vi "step.util.flag-matching.vi"(6 "include step flags":bool=TRUE, 9 "stepElement":variant, 10 "procElement":variant, 11 "$string in":string="$module $proc $step $clk $date_$time ") -> (3 "formated string out":string="myModule myProc myStep 3800935574.524293 2024-06-11_10-26-15 ")   [LabVIEW 2024]
uses:
  controls/typeProcVarientName.ctl
  controls/typeStepVarients.ctl
  Polymorphics/variantCtrlString.vi
  Polymorphics/variantCtrlNumber.vi
  proc.util.validateParamExist.vi
  <vilib>/Utility/error.llb/Clear Errors.vi
  <vilib>/Utility/error.llb/Trim Whitespace One-Sided.vi
  globals/globals-engine.vi
  util.error.create.vi
  <vilib>/Utility/libraryn.llb/Create Directory Recursive.vi
panel:
  out "array out":string[](array[string])
  in  "time stamp":timestamp
  # "this vi should support matching fields file and io node names"
  # "$date\n$timestamp"
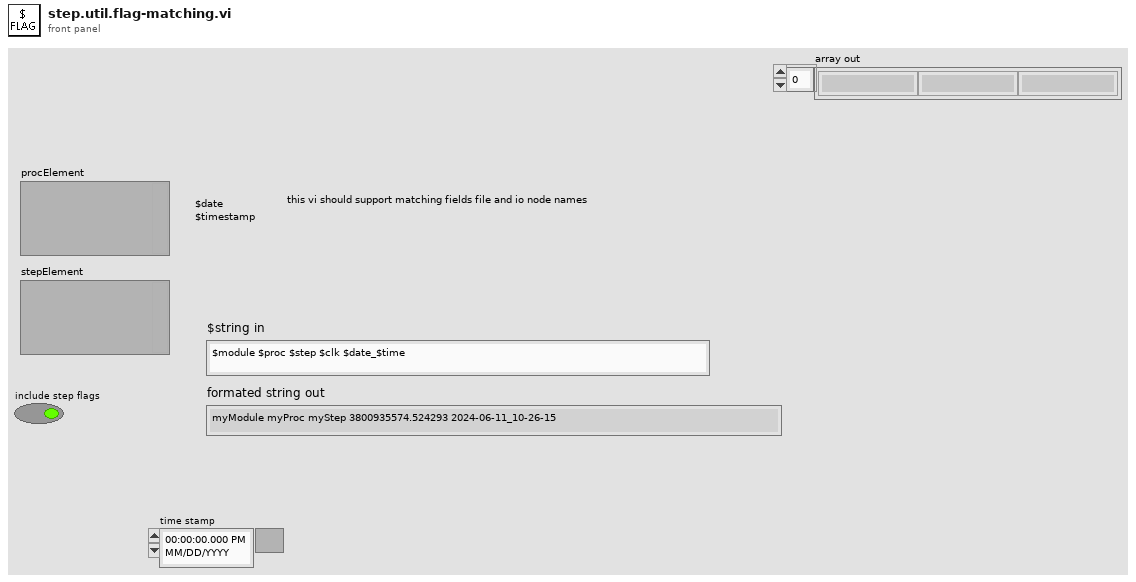
[diagram p1: front panel]
types:
  T1 = typedef "typeStepVarients.ctl" = enum16{"stepNameID", "stepFunction", "stepReport", "stepSetpoint", "stepPointer", "stepProcPointer", "stepIoPointer", "stepIoValue", "stepFilePointer", "stepMessage", "stepTimeString", "stepNumReg", "stepStrReg", "stepSeconds", "stepUnitDoseParams", "stepUnitIndex"}
  T2 = typedef "typeProcVarientName.ctl" = enum16{"procNameID", "procModuleID", "procPath", "procIsRunning", "procIndex", "procModule", "procRegisterNumeric", "procRegisterString", "procReport", "procReportPrev", "procCLK", "procStepPointer", "procType"}
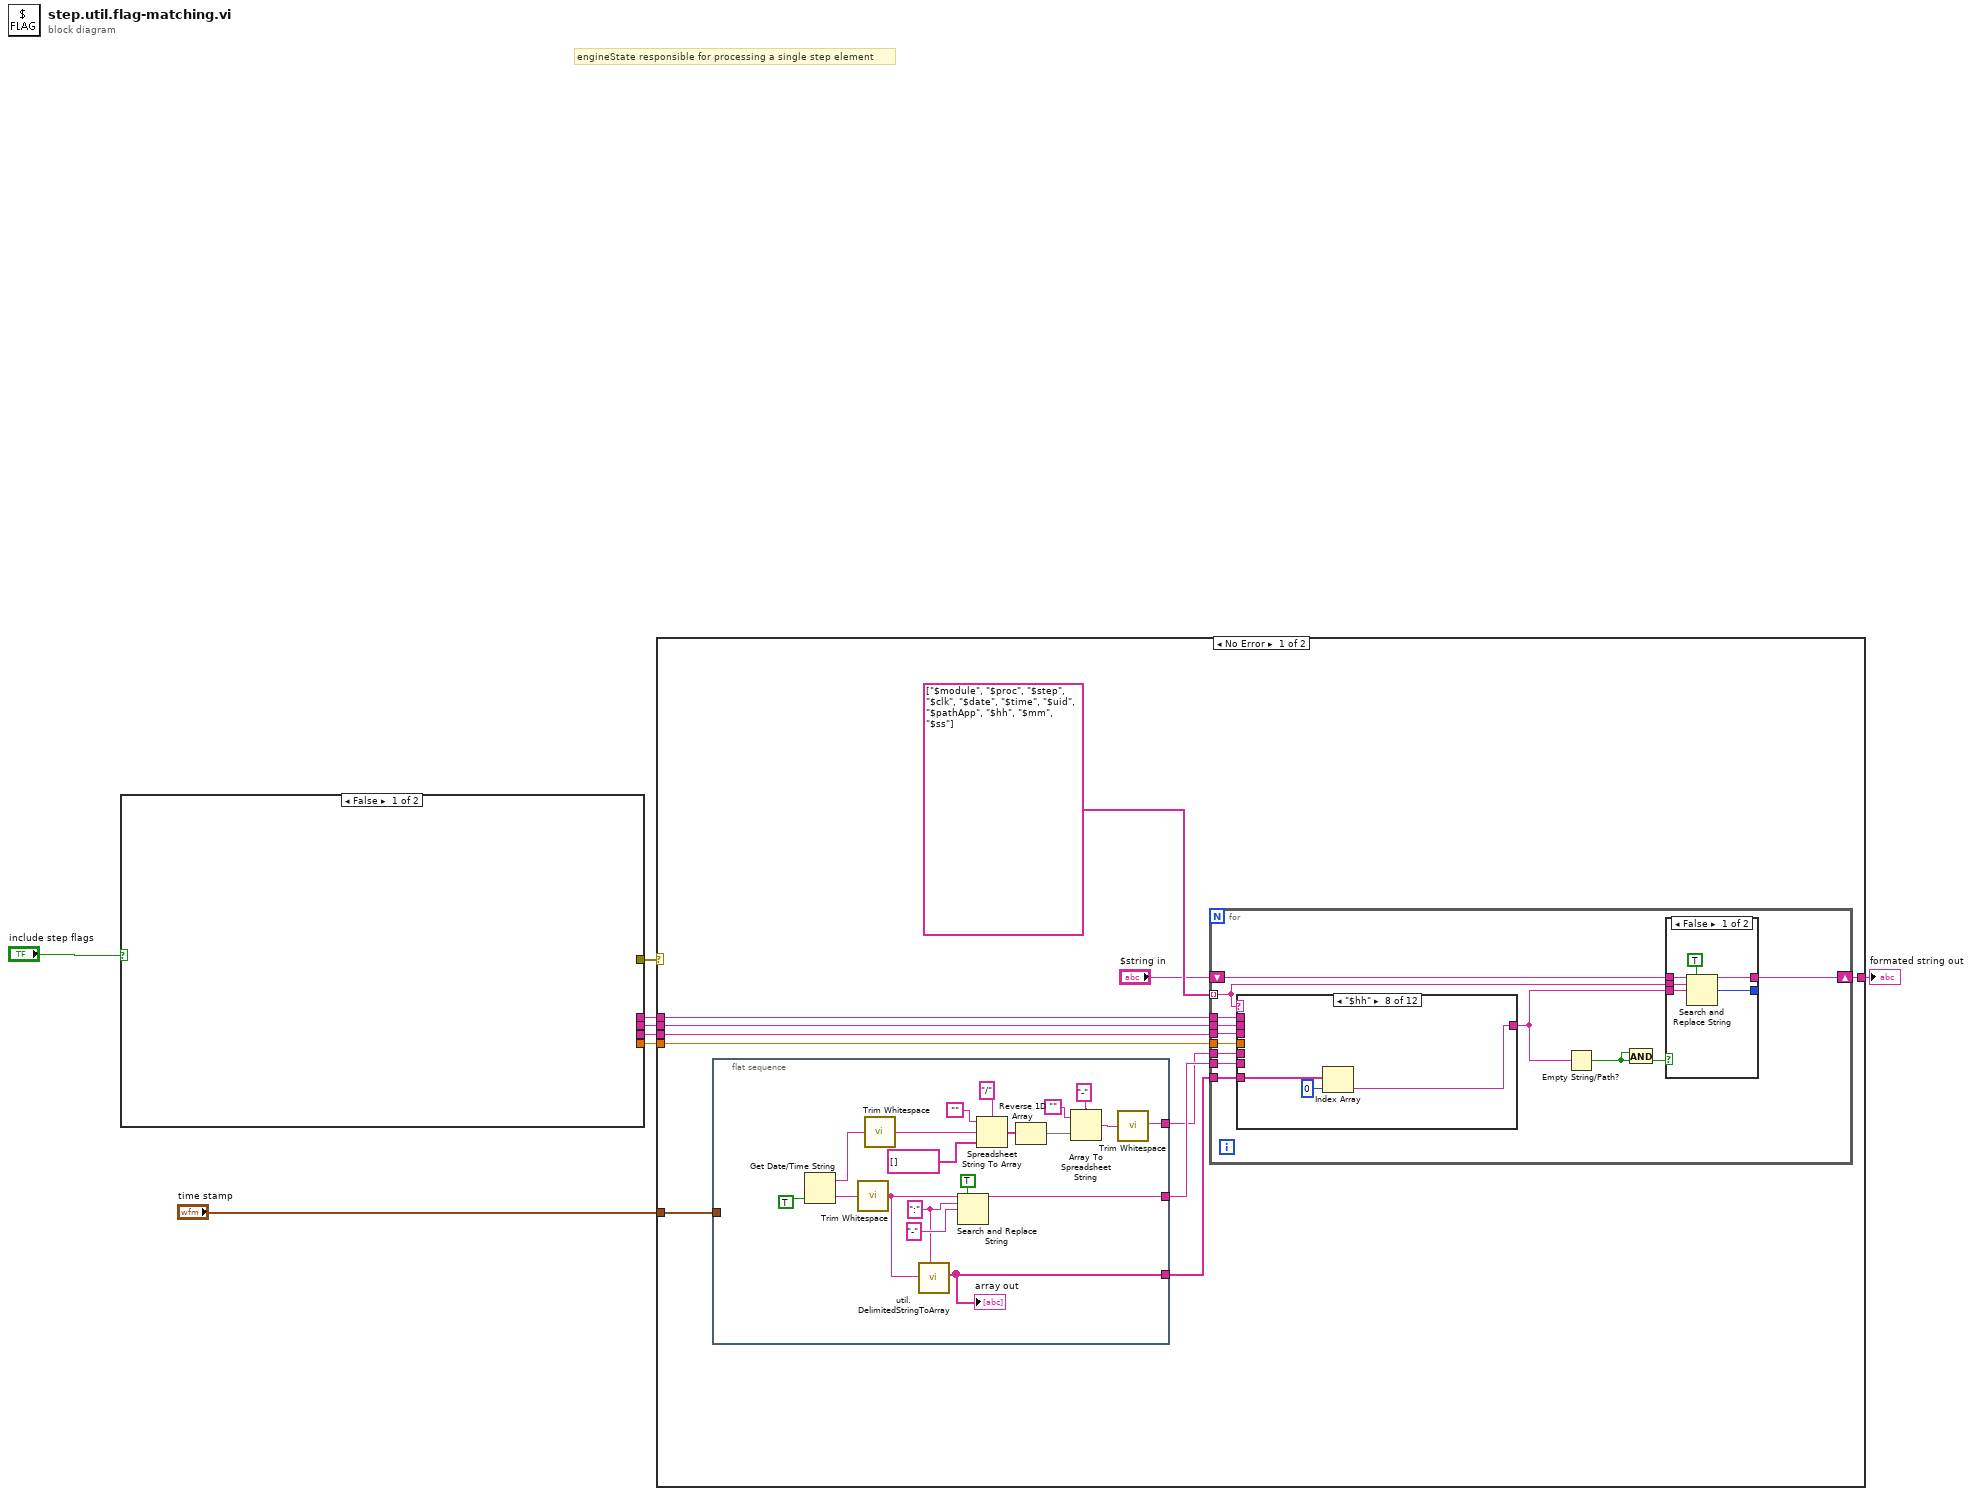
[diagram p0: block diagram]
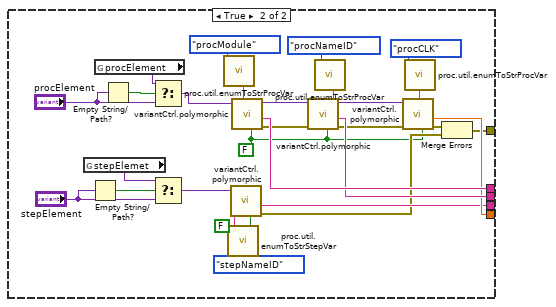
[diagram p2: hidden frame]
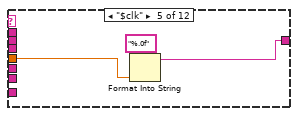
[diagram p8: hidden frame]
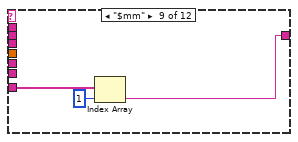
[diagram p11: hidden frame]
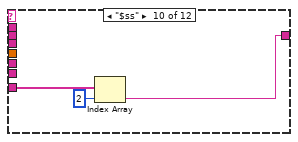
[diagram p12: hidden frame]
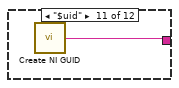
[diagram p13: hidden frame]
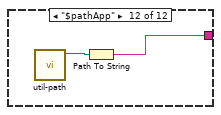
[diagram p14: hidden frame]
diagram:
  # "engineState responsible for processing a single step element"
  n1 = case shown="False" "include step flags" {
    tunnel: [_ w25] -> w7
    tunnel: [_ w24] -> w6
    tunnel: [_ w23] -> w5
    tunnel: [_ w20] -> w4
    tunnel: [_ w11] -> w3
    frame False {
    }
    frame True {
      w9 = FALSE ("isRequired (T)")
      n2 = global read "globals-engine.vi" "stepElemet"() -> (w36:variant)
      n3 = Empty String/Path?(string/path="stepElement") -> (empty?=w15:bool)
      n4 = global read "globals-engine.vi" "procElement"() -> (w37:variant)
      n5 = Empty String/Path?(string/path="procElement") -> (empty?=w17:bool)
      n6 = Select(t=w37, s=w17, f="procElement") -> (s? t:f=w33:variant)
      n7 = Select(t=w36, s=w15, f="stepElement") -> (s? t:f=w35:variant)
      n8 = call "proc.util.enumToStrProcVar.vi"("Proc var"=typeProcVarientName."procModule" ("proc var")) -> ("String"=w31:string)  [unwired: 10 in]
      n9 = call "proc.util.enumToStrStepVar.vi"("Step var"=typeStepVarients."stepNameID" ("proc var")) -> ("String"=w22:string)  [unwired: 10 in]
      n10 = call-poly "variantCtrl.polymorphic.vi"("isRequired (T)"=FALSE, "name in"=w22, "Step in"=w35) -> ("error out"=w12:errorcluster, "String Value"=w20:string)  [unwired: 5 in, 2 out]
      n11 = call-poly "variantCtrl.polymorphic.vi"("isRequired (T)"=w9, "name in"=w31, "Step in"=w33) -> ("error out"=w13:errorcluster, "String Value"=w25:string, "Step out"=w32:variant)  [unwired: 5 in, 1 out]
      n12 = call "proc.util.enumToStrProcVar.vi"("Proc var"=typeProcVarientName."procNameID" ("proc var")) -> ("String"=w28:string)  [unwired: 10 in]
      n13 = call-poly "variantCtrl.polymorphic.vi"("isRequired (T)"=w9, "error in"=w13, "name in"=w28, "Step in"=w32) -> ("error out"=w14:errorcluster, "String Value"=w24:string, "Step out"=w34:variant)  [unwired: 4 in, 1 out]
      n14 = call "proc.util.enumToStrProcVar.vi"("Proc var"=typeProcVarientName."procCLK" ("proc var")) -> ("String"=w27:string)  [unwired: 10 in]
      n15 = call-poly "variantCtrl.polymorphic.vi"("isRequired (T)"=w9, "error in"=w14, "name in"=w27, "variant in"=w34) -> ("error out"=w10:errorcluster, "number"=w23:dbl)  [unwired: 4 in, 2 out]
      n16 = Merge Errors(w10, w12) -> (w11:errorcluster)
    }
  }
  n17 = case shown="No Error" w3 {
    tunnel: [w46 _] -> w8
    tunnel: w7 -> [w43 _]
    tunnel: w6 -> [w42 _]
    tunnel: w5 -> [w41 _]
    tunnel: w4 -> [w40 _]
    tunnel: "time stamp" -> [w39 _]
    frame No Error {
      n18 = flat-sequence {
        tunnel: [w94] -> w45
        tunnel: [w92] -> w44
        tunnel: w39 -> [_]
        tunnel: [w89] -> w38
        frame #0 {
          w90 = ":" ("search string")
          n19 = Get Date/Time String(want seconds? (F)=TRUE) -> (date string=w97:string, time string=w95:string)  [unwired: 2 in]
          n20 = call <vilib>:"Trim Whitespace.vi"("string"=w95) -> ("trimmed string"=w91:string)  [unwired: 1 in]
          n21 = call <vilib>:"Trim Whitespace.vi"("string"=w97) -> ("trimmed string"=w93:string)  [unwired: 1 in]
          n22 = call "util.DelimitedStringToArray.vi"("delimiter (,)"=w90, "delimitaed string"=w91) -> ("array out"=w89:string[])  [unwired: 9 in]
          "array out" <- w89
          n23 = Search and Replace String(replace all?=TRUE ("replace all? (F)"), input string=w91, search string=w90, replace string="-" ("search string")) -> (result string=w94:string)  [unwired: 4 in, 3 out]
          n24 = Spreadsheet String To Array(delimiter (Tab)="/", format string="" ("delimiter (Tab)"), spreadsheet string=w93, array type (2D Dbl)=string[] []) -> (array=w104:string[])
          n25 = Reverse 1D Array(array=w104) -> (reversed array=w103:string[])
          n26 = Array To Spreadsheet String(delimiter (Tab)="-", array=w103, 3:"" ("format string")) -> (spreadsheet string=w96:string)
          n27 = call <vilib>:"Trim Whitespace.vi"("string"=w96) -> ("trimmed string"=w92:string)  [unwired: 1 in]
        }
      }
      n28 = for {
        tunnel: string[] ["$module", "$proc", "$step", "$clk", "$date", "$time", "$uid", "$pathApp", "$hh", "$mm", "$ss"] -> [w60] mode=indexing
        tunnel: w43 -> [w59]
        tunnel: w42 -> [w61]
        tunnel: w40 -> [w58]
        tunnel: w41 -> [w57]
        tunnel: w44 -> [w56]
        tunnel: w45 -> [w55]
        shift-right: [w54] -> w46
        shift-left: "$string in" -> [w53]
        tunnel: w38 -> [w49]
        n29 = case shown="\"$hh\"" w60 {
          tunnel: w61 -> [_ _ w70 _ _ _ _ _ _ _ _ _]
          tunnel: [_ w69 w70 w71 w73 w75 w76 w78 w81 w84 w86 w88] -> w52
          tunnel: w59 -> [_ w69 _ _ _ _ _ _ _ _ _ _]
          tunnel: w58 -> [_ _ _ w71 _ _ _ _ _ _ _ _]
          tunnel: w57 -> [_ _ _ _ w74 _ _ _ _ _ _ _]
          tunnel: w56 -> [_ _ _ _ _ w75 _ _ _ _ _ _]
          tunnel: w55 -> [_ _ _ _ _ _ w76 _ _ _ _ _]
          tunnel: w49 -> [_ _ _ _ _ _ _ w79 w82 w85 _ _]
          frame Default {
          }
          frame "$module" {
          }
          frame "$proc" {
          }
          frame "$step" {
          }
          frame "$clk" {
            n30 = Format Into String(format string="%.0f", w74) -> (resulting string=w73:string)  [unwired: 2 in, 1 out]
          }
          frame "$date" {
          }
          frame "$time" {
          }
          frame "$hh" {
            n31 = Index Array(array=w79, index=0) -> (element=w78:string)
          }
          frame "$mm" {
            n32 = Index Array(array=w82, index=1) -> (element=w81:string)
          }
          frame "$ss" {
            n33 = Index Array(array=w85, index=2) -> (element=w84:string)
          }
          frame "$uid" {
            n34 = call <vilib>:"Create NI GUID.vi"() -> ("NI GUID"=w86:string)
          }
          frame "$pathApp" {
            n35 = call "util-path.vi"() -> ("AppPath"=w87:path)  [unwired: 7 in, 4 out]
            n36 = Path To String(path=w87) -> (string=w88:string)
          }
        }
        n37 = Empty String/Path?(string/path=w52) -> (empty?=w50:bool)
        n38 = And(x=w50, y=w50) -> (x .and. y?=w51:bool)
        n39 = case shown="False" w51 {
          tunnel: w53 -> [w67 w68]
          tunnel: w60 -> [w66 _]
          tunnel: w52 -> [w65 _]
          tunnel: [w63 w68] -> w54
          tunnel: [w62 _] -> _
          frame False {
            # "not empty"
            n40 = Search and Replace String(replace all?=TRUE ("replace all? (F)"), input string=w67, search string=w66, replace string=w65) -> (result string=w63:string, number of replacements=w62:i32)  [unwired: 4 in, 2 out]
          }
          frame True {
          }
        }
      }
    }
    frame Error {
    }
  }
  "formated string out" <- w8
